vi "DENSITY.vi"(0 "DoseStrokes":i32=20, 1 "uL/stroke":i32=6, 5 "GUID":string, 9 "PrimeStrokes":i32=20, 11 "PrimeStrokes2":i32=3) -> (3 "density (g/mL)":dbl, 4 "mean":dbl format="%0.4f", 6 "mean 2":dbl format="%0.4f", 8 "standard deviation":dbl format="%0.4f", 10 "standard deviation 2":dbl format="%0.4f", 14 "xxx":bool[](array[boolean]), 15 "Err?":string)   [LabVIEW 2019]
uses:
  <vilib>/Analysis/NI_AALBase.lvlib
panel:
  out "sample (g)":dbl[](array[numeric])
  out "variance 2":dbl format="%0.4f"
  out "InvalidCommandErr? 2":bool
  out "tare (g)":dbl[](array[numeric])
  out "variance":dbl format="%0.4f"
  out "InvalidCommandErr?":bool
  out "log_string":string
  out "SampleVolume (mL)":dbl
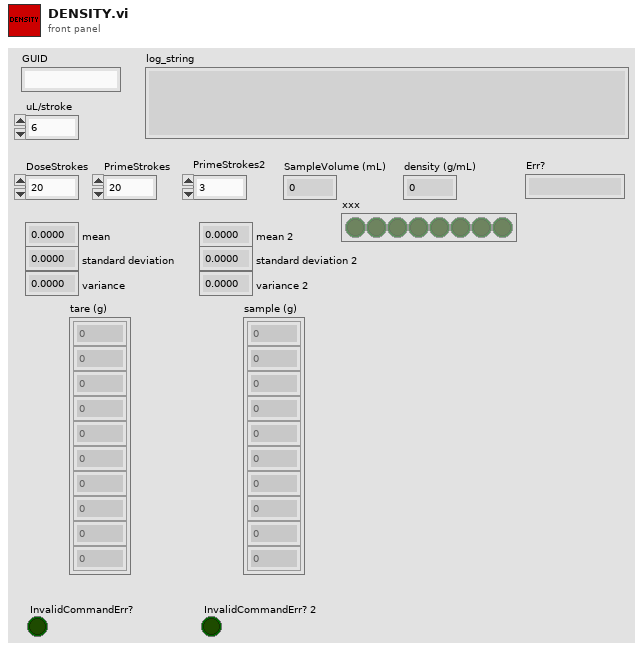
[diagram p1: front panel]
types:
  T1 = enum16{"open", "replace", "create", "open or create", "replace or create", "replace or create with confirmation"}
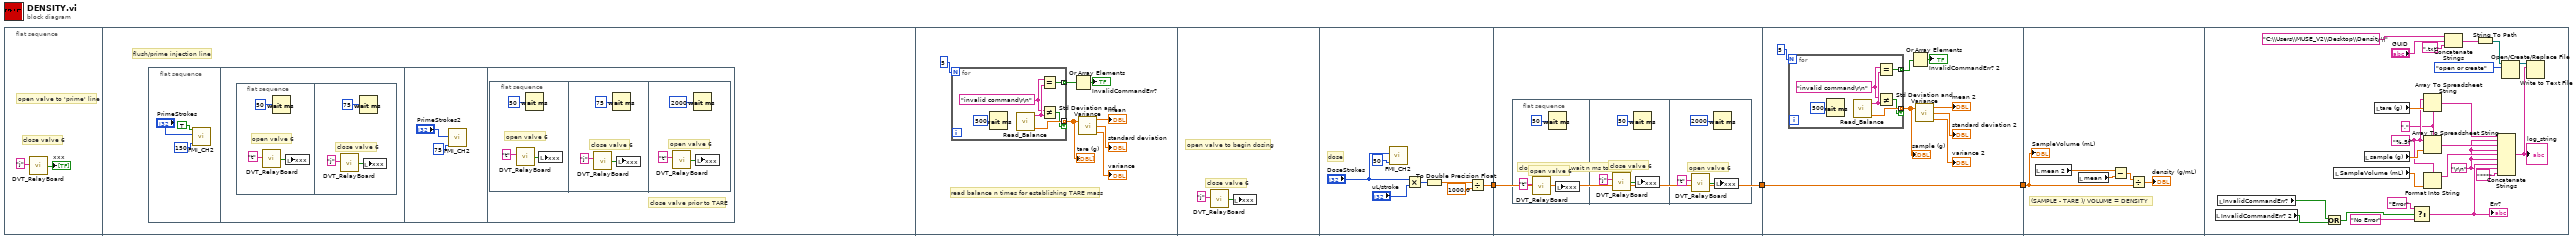
[diagram p0: block diagram]
diagram:
  n1 = flat-sequence {
    tunnel: [w47] -> w2
    tunnel: [w48] -> w1
    tunnel: w2 -> [w48]
    tunnel: [w65] -> w3
    tunnel: w1 -> [w65]
    tunnel: w3 -> [w73]
    frame #0 {
      # "close valve 6"
      # "open valve to 'prime' line"
      n2 = call "DVT_RelayBoard.vi"("write buffer"="j") -> ("Boolean array"=→"xxx":bool[])  [unwired: 3 in, 2 out]
    }
    frame #1 {
      # "flush/prime injection line"
      n3 = flat-sequence {
        frame #0 {
          n4 = call "FMI_CH2.vi"("RPM"=150, "Strokes"="PrimeStrokes", "Home Pump"=TRUE) -> ()  [unwired: 5 in]
        }
        frame #1 {
          n5 = flat-sequence {
            frame #0 {
              # "open valve 6"
              n6 = call "DVT_RelayBoard.vi"("write buffer"="t") -> ("Boolean array"=w9:bool[])  [unwired: 3 in, 2 out]
              n7 = Wait (ms)(milliseconds to wait=u32 50) -> ()  [unwired: 1 out]
              n8 = local write "xxx"(w9) -> ()
            }
            frame #1 {
              # "close valve 6"
              n9 = call "DVT_RelayBoard.vi"("write buffer"="j") -> ("Boolean array"=w13:bool[])  [unwired: 3 in, 2 out]
              n10 = Wait (ms)(milliseconds to wait=u32 75) -> ()  [unwired: 1 out]
              n11 = local write "xxx"(w13) -> ()
            }
          }
        }
        frame #2 {
          n12 = call "FMI_CH2.vi"("RPM"=75, "Strokes"="PrimeStrokes2") -> ()  [unwired: 6 in]
        }
        frame #3 {
          # "close valve prior to TARE"
          n13 = flat-sequence {
            frame #0 {
              # "open valve 6"
              n14 = call "DVT_RelayBoard.vi"("write buffer"="t") -> ("Boolean array"=w17:bool[])  [unwired: 3 in, 2 out]
              n15 = Wait (ms)(milliseconds to wait=u32 50) -> ()  [unwired: 1 out]
              n16 = local write "xxx"(w17) -> ()
            }
            frame #1 {
              # "close valve 6"
              n17 = call "DVT_RelayBoard.vi"("write buffer"="j") -> ("Boolean array"=w21:bool[])  [unwired: 3 in, 2 out]
              n18 = Wait (ms)(milliseconds to wait=u32 75) -> ()  [unwired: 1 out]
              n19 = local write "xxx"(w21) -> ()
            }
            frame #2 {
              # "open valve 6"
              n20 = call "DVT_RelayBoard.vi"("write buffer"="t") -> ("Boolean array"=w23:bool[])  [unwired: 3 in, 2 out]
              n21 = Wait (ms)(milliseconds to wait=u32 2000) -> ()  [unwired: 1 out]
              n22 = local write "xxx"(w23) -> ()
            }
          }
        }
      }
    }
    frame #2 {
      # "read balance n times for establishing TARE mass"
      n23 = for {
        N: 5 -> [_]
        tunnel: [w37] -> w32 mode=indexing if=w34
        tunnel: [w33] -> w30 mode=indexing
        w35 = "invalid command\r\n"
        n24 = Wait (ms)(milliseconds to wait=u32 500) -> ()  [unwired: 1 out]
        n25 = call "Read_Balance.vi"() -> ("dbl"=w37:dbl, "string"=w36:string)  [unwired: 4 in]
        n26 = Equal?(x=w35, y=w36) -> (x = y?=w33:bool)
        n27 = Not Equal?(x=w35, y=w36) -> (x != y?=w34:bool)
      }
      "tare (g)" <- w32
      n28 = Or Array Elements(Boolean array=w30) -> (logical OR=→"InvalidCommandErr?":bool)
      n29 = call <vilib>:"Std Deviation and Variance.vi"("X"=w32) -> ("mean"=→"mean":dbl, "standard deviation"=→"standard deviation":dbl, "variance"=→"variance":dbl)  [unwired: 1 in]
    }
    frame #3 {
      # "close valve 6"
      # "open valve to begin dosing"
      n30 = call "DVT_RelayBoard.vi"("write buffer"="j") -> ("Boolean array"=w39:bool[])  [unwired: 3 in, 2 out]
      n31 = local write "xxx"(w39) -> ()
    }
    frame #4 {
      # "dose"
      n32 = call "FMI_CH2.vi"("RPM"=50, "Strokes"="DoseStrokes") -> ()  [unwired: 6 in]
      n33 = Multiply(x="DoseStrokes", y="uL/stroke") -> (x*y=w41:i32)
      n34 = To Double Precision Float(number=w41) -> (double precision float=w42:dbl)
      n35 = Divide(x=w42, y=1000.0) -> (x/y=w47:dbl)
    }
    frame #5 {
      # "close valve and wait n ms to stabilize"
      n36 = flat-sequence {
        frame #0 {
          # "open valve 6"
          n37 = call "DVT_RelayBoard.vi"("write buffer"="t") -> ("Boolean array"=w50:bool[])  [unwired: 3 in, 2 out]
          n38 = Wait (ms)(milliseconds to wait=u32 50) -> ()  [unwired: 1 out]
          n39 = local write "xxx"(w50) -> ()
        }
        frame #1 {
          # "close valve 6"
          n40 = call "DVT_RelayBoard.vi"("write buffer"="j") -> ("Boolean array"=w53:bool[])  [unwired: 3 in, 2 out]
          n41 = Wait (ms)(milliseconds to wait=u32 50) -> ()  [unwired: 1 out]
          n42 = local write "xxx"(w53) -> ()
        }
        frame #2 {
          # "open valve 6"
          n43 = call "DVT_RelayBoard.vi"("write buffer"="t") -> ("Boolean array"=w55:bool[])  [unwired: 3 in, 2 out]
          n44 = Wait (ms)(milliseconds to wait=u32 2000) -> ()  [unwired: 1 out]
          n45 = local write "xxx"(w55) -> ()
        }
      }
    }
    frame #6 {
      n46 = for {
        N: 5 -> [_]
        tunnel: [w70] -> w64 mode=indexing if=w67
        tunnel: [w66] -> w62 mode=indexing
        w68 = "invalid command\r\n"
        n47 = Wait (ms)(milliseconds to wait=u32 500) -> ()  [unwired: 1 out]
        n48 = call "Read_Balance.vi"() -> ("dbl"=w70:dbl, "string"=w69:string)  [unwired: 4 in]
        n49 = Equal?(x=w68, y=w69) -> (x = y?=w66:bool)
        n50 = Not Equal?(x=w68, y=w69) -> (x != y?=w67:bool)
      }
      "sample (g)" <- w64
      n51 = Or Array Elements(Boolean array=w62) -> (logical OR=→"InvalidCommandErr? 2":bool)
      n52 = call <vilib>:"Std Deviation and Variance.vi"("X"=w64) -> ("mean"=→"mean 2":dbl, "standard deviation"=→"standard deviation 2":dbl, "variance"=→"variance 2":dbl)  [unwired: 1 in]
    }
    frame #7 {
      # "(SAMPLE - TARE )/ VOLUME = DENSITY"
      n53 = local read "mean 2"() -> (w76:dbl)
      n54 = local read "mean"() -> (w75:dbl)
      n55 = Subtract(x=w76, y=w75) -> (x-y=w74:dbl)
      n56 = Divide(x=w74, y=w73) -> (x/y=→"density (g/mL)":dbl)
      "SampleVolume (mL)" <- w73
    }
    frame #8 {
      w79 = "\r\n"
      w85 = "," ("delimiter (Tab)")
      w86 = "%.5f" ("format (%.3f)")
      n57 = local read "InvalidCommandErr? 2"() -> (w78:bool)
      n58 = local read "InvalidCommandErr?"() -> (w77:bool)
      n59 = Or(x=w77, y=w78) -> (x .or. y?=w80:bool)
      n60 = local read "SampleVolume (mL)"() -> (w90:dbl)
      n61 = local read "sample (g)"() -> (w91:dbl[])
      n62 = local read "tare (g)"() -> (w93:dbl[])
      n63 = Select(t="Error" ("string"), s=w80, f="No Error") -> (s? t:f=w83:string)
      "Err?" <- w83
      n64 = Array To Spreadsheet String(delimiter (Tab)=w85, array=w93, 3:w86) -> (spreadsheet string=w92:string)
      n65 = Array To Spreadsheet String(delimiter (Tab)=w85, array=w91, 3:w86) -> (spreadsheet string=w89:string)
      n66 = Format Into String(format string=w86, w90) -> (resulting string=w88:string)  [unwired: 2 in, 1 out]
      n67 = Concatenate Strings("C:\\Users\\MUSE_V2\\Desktop\\Density\\", "GUID", ".txt" ("string")) -> (w98:string)
      n68 = String To Path(string=w98) -> (path=w96:path)
      n69 = Concatenate Strings(w92, w79, w89, w79, w88, w79, w83, w79, "***" ("string")) -> (w87:string)
      "log_string" <- w87
      n70 = Open/Create/Replace File(file path (use dialog)=w96, operation (0:open)=T1."open or create") -> (refnum out=w97:refnum<file>)  [unwired: 4 in, 2 out]
      n71 = Write to Text File(file (use dialog)=w97, text=w87) -> ()  [unwired: 2 in, 3 out]
    }
  }
